vi "C1G2_Assemble smallQuery.vi"(7 "Symbol Rate":dbl=10000000.0 format="%#_6p", 9 "Parameters Query":T2={"DR"=FALSE, "M"=1, "TRext (T=Pilot Tone)"=FALSE, "Sel"=1, "Session"=0, "Q"=0, "Target"=FALSE} {"Session" items=["S0", "S1", "S2", "S3"]; "Sel" items=["All", "All2", "~SL", "SL"]; "M" items=["M=1", "M=2", "M=4", "M=8"]}, 11 "Parameters Symbols":T1={"Tari"=8e-06, "PW"=0.5, "factor for \"1\" symbol"=0.5, "RTcal"=2.5, "TRcal"=3.0, "Delimiter"=1.25e-05} {"TRcal" min=1.1 max=3.0 step=0.1; "RTcal" min=2.5 max=3.0 step=0.1; "factor for \"1\" symbol" min=0.5 max=1.0 step=0.1; "PW" min=0.265 max=0.525 step=0.001; "Tari" format="%#_3p"}) -> (2 "Signal out":u8[](array[numeric]))   [LabVIEW 2015]
panel:
  out "Symbols Query":i32
  out "Symbols All":i32=53374
  out "Digital Waveform":waveform(u8)(graph)={"t0"=timestamp(0 s since 1904-01-01), "dt"=1e-07, "Y"=array[53374 elements]}
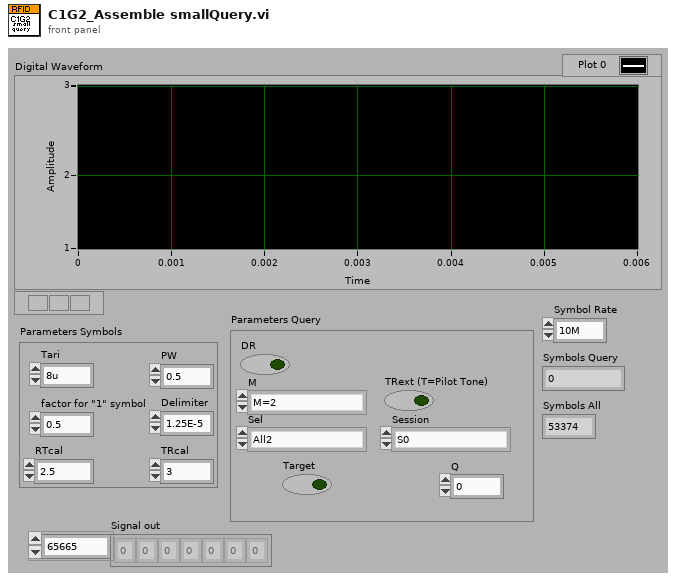
[diagram p1: front panel]
types:
  T1 = cluster{"Tari":dbl, "PW":dbl, "factor for \"1\" symbol":dbl, "RTcal":dbl, "TRcal":dbl, "Delimiter":dbl}
  T2 = cluster{"DR":bool, "M":u16, "TRext (T=Pilot Tone)":bool, "Sel":u16, "Session":u16, "Q":u8, "Target":bool}
  T3 = typedef "C1G2_BasicsData.ctl" = cluster{"Symbol \"0\"":u8[], "Symbol \"1\"":u8[], "RT Preamble":u8[], "RT Frame Sync":u8[], "Sample Rate":dbl, "LOW-Pulse":u8[], "HIGH-Pulse":u8[], "RT cal":u8[]}
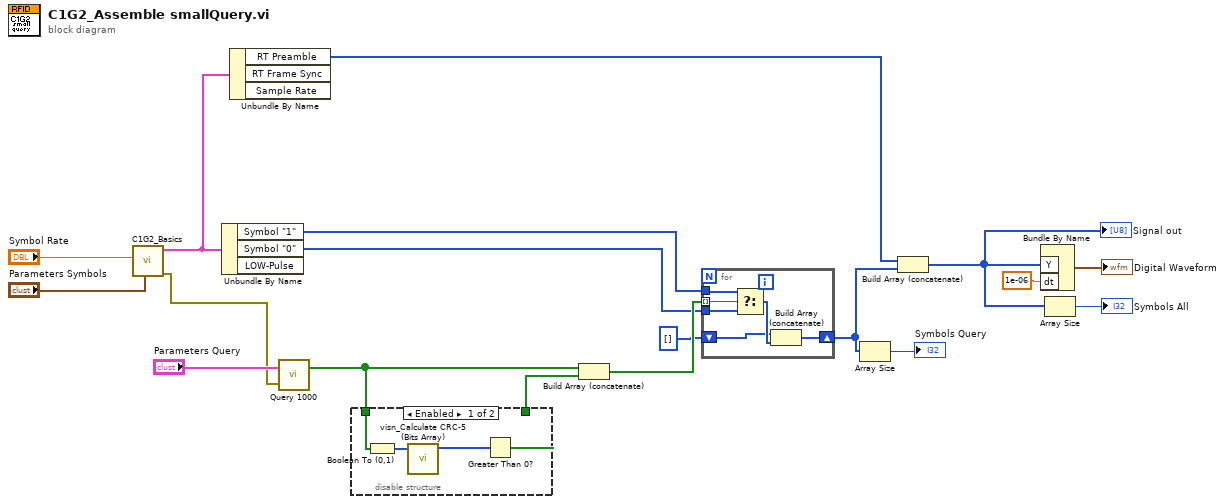
[diagram p0: block diagram]
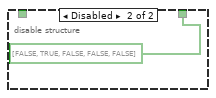
[diagram p2: hidden frame]
diagram:
  n1 = call "C1G2_Basics.vi"("Parameters Symbols"="Parameters Symbols", "Symbol Rate"="Symbol Rate") -> ("error out"=w1:errorcluster, "Basic Components"=w12:T3)  [unwired: 8 in]
  n2 = Unbundle By Name(w12) -> ("Symbol \"1\""=w9:u8[], "Symbol \"0\""=w8:u8[])  [unwired: 1 out]
  n3 = Unbundle By Name(w12) -> ("RT Preamble"=w4:u8[])  [unwired: 2 out]
  n4 = call "Query 1000.vi"("error in (no error)"=w1, "Parameters Query"="Parameters Query") -> ("Array"=w5:bool[])  [unwired: 1 out]
  n5 = disable-structure shown="Enabled" {
    disable-tunnel: w5 -> [w21 _]
    disable-tunnel: [w19 bool[] [FALSE, TRUE, FALSE, FALSE, FALSE]] -> w11
    frame Enabled {
      n6 = Boolean To (0,1)(Boolean=w21) -> (0, 1=w22:i16[])
      n7 = call "visn_Calculate CRC-5 (Bits Array).vi"("Bits Array"=w22) -> ("CRC-5"=w20:u8[])  [unwired: 10 in]
      n8 = Greater Than 0?(x=w20) -> (x > 0?=w19:bool[])
    }
    frame Disabled {
    }
  }
  n9 = Build Array (concatenate)(w5, w11) -> (w10:bool[])
  n10 = for {
    tunnel: w10 -> [w29] mode=indexing
    tunnel: w8 -> [w27]
    tunnel: w9 -> [w28]
    shift-right: [w26] -> w3
    shift-left: u8[] [] ("s? t:f") -> [w24]
    n11 = Select(t=w28, s=w29, f=w27) -> (s? t:f=w25:u8[])
    n12 = Build Array (concatenate)(w24, w25) -> (w26:u8[])
  }
  n13 = Array Size(array=w3) -> (size(s)=→"Symbols Query":i32)
  n14 = Build Array (concatenate)(w4, w3) -> (w2:u8[])
  "Signal out" <- w2
  n15 = Bundle By Name("Y"=w2, "dt"=1e-06) -> (→"Digital Waveform":waveform(u8))  [unwired: 1 in]
  n16 = Array Size(array=w2) -> (size(s)=→"Symbols All":i32)
